vi "DAQmx Simulator.vi"() -> (0 "Analog Input":dbl format="%#.1g")   [LabVIEW 2023]
uses:
  <vilib>/numeric/Random Number (Range) DBL.vi
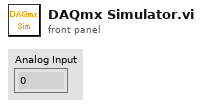
[diagram p1: front panel]
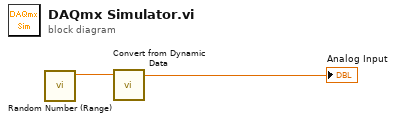
[diagram p0: block diagram]
diagram:
  n1 = call-poly <vilib>:"Random Number (Range).vi"() -> ("number"=w2:dbl)  [unwired: 11 in]
  n2 = call "Convert from Dynamic Data"("Dynamic Data Type"=w2) -> ("Scalar"=→"Analog Input":dbl)  [unwired: 3 in]
